vi "GetIndexFromItem.vi"(8 "error in (no error)":errorcluster, 10 "Item Name":string, 11 "MenuCol in":refnum<class "MenuCol.lvclass">) -> (0 "error out":errorcluster, 1 "Item Exists":bool, 2 "Item Index":i32, 3 "MenuCol out":refnum<class "MenuCol.lvclass">)   [LabVIEW 2013, in "MenuCol.lvclass"]
uses:
  MenuCol.lvclass
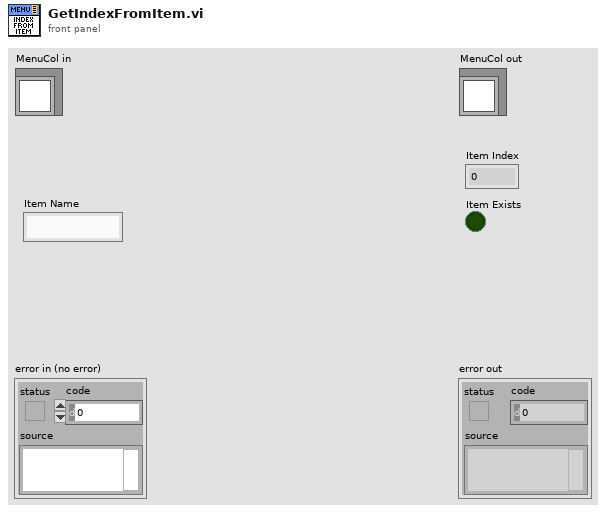
[diagram p1: front panel]
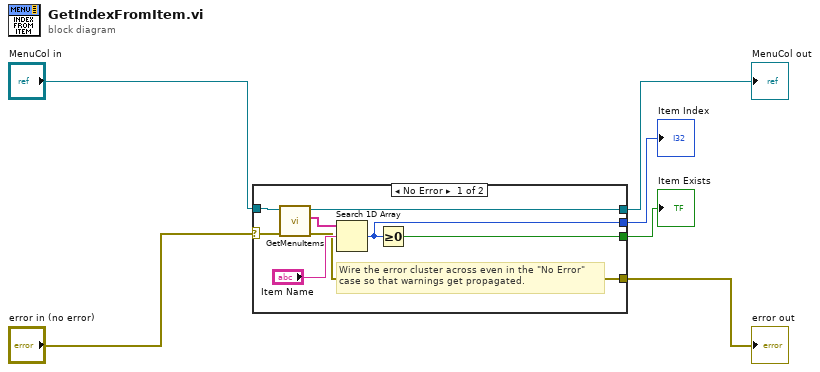
[diagram p0: block diagram]
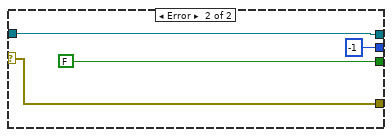
[diagram p2: hidden frame]
diagram:
  n1 = case shown="No Error" "error in (no error)" {
    selector: "error in (no error)" -> [w12 w18]
    tunnel: [w10 w18] -> w1
    tunnel: [w13 w17] -> w2
    tunnel: "MenuCol in" -> [w14 w17]
    tunnel: [w9 -1 ("index of element")] -> w5
    tunnel: [w8 FALSE] -> w6
    frame No Error {
      # "Wire the error cluster across even in the \"No Error\"\ncase so that warnings get propagated."
      n2 = call-dynamic "GetMenuItems.vi"("error in (no error)"=w12, "MenuCol in"=w14) -> ("error out"=w10:errorcluster, "MenuLabels"=w7:string[], "MenuCol out"=w13:refnum<class "MenuCol.lvclass">)  [unwired: 6 in, 1 out]
      n3 = Search 1D Array(1D array=w7, element="Item Name") -> (index of element=w9:i32)  [unwired: 1 in]
      n4 = Greater Or Equal To 0?(x=w9) -> (x >= 0?=w8:bool)
    }
    frame Error {
    }
  }
  "error out" <- w1
  "MenuCol out" <- w2
  "Item Exists" <- w6
  "Item Index" <- w5
